vi "simple PID.vi"(4 "lower limit":dbl format="%.2f", 6 "upper limit":dbl format="%.2f", 7 "process variable":dbl format="%.2f", 8 "D":dbl=0.05 format="%.2f", 9 "I":dbl=0.1 format="%.2f", 10 "P":dbl=1.0 format="%.2f", 11 "set point":dbl format="%.2f") -> (3 "output value":dbl format="%.2f")   [LabVIEW 2016]
doc: "This is a simple PID which can be used to control a system. The idea of a PID is to control a system by comparing the set point (the system value you want) to the process variable (the current system value), and adjusting the output value (what you output to the system in an attempt to get the process variable to approach the set point.\n\nThe set point is the value you desire the system to achieve.\n\nThe process variable is the current value of your system, and is usually acquired by an analog input channel of your DAQ device.\n\nP is the Proportional component. This is the amount by which the error gets multiplied. The error is the set point minus the process variable.\n\nI is the Integral component. This is how much the PID output will depend on what has happened in the past.\n\nD is the derivative component. This is how much the PID output will depend on speculation of what will happen in the future.\n\nThe output value is the PID output which is usually generated at an analog output channel of your DAQ device in an attempt to get the process variable equal to the set point.\n\nThe upper limit is the maximum value the PID can output to the system.\n\nThe lower limit is the minimum value the PID can output to the system."
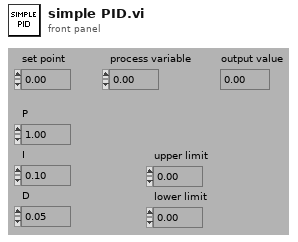
[diagram p1: front panel]
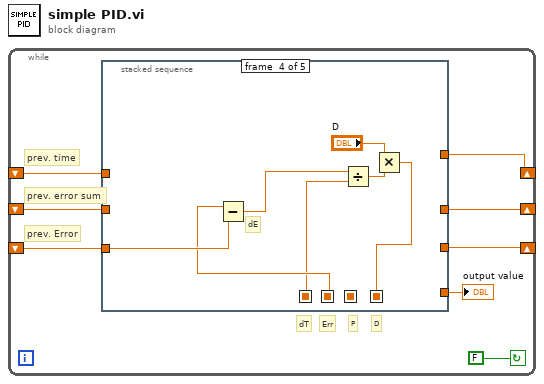
[diagram p0: block diagram]
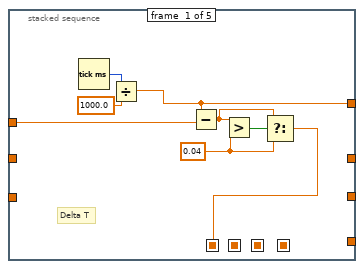
[diagram p2: hidden frame]
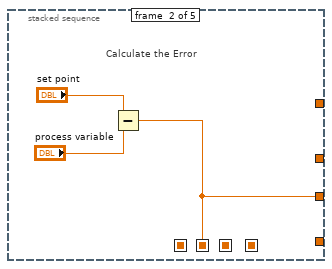
[diagram p3: hidden frame]
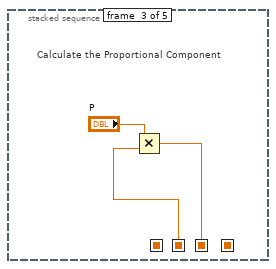
[diagram p4: hidden frame]
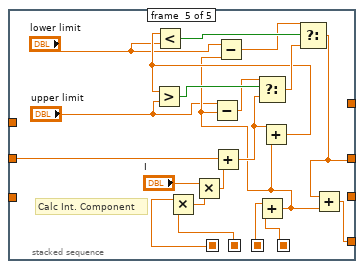
[diagram p5: hidden frame]
diagram:
  n1 = while {
    shift-left: _ -> [w3]
    shift-right: [w4] -> _
    shift-left: _ -> [w6]
    shift-right: [w5] -> _
    shift-left: _ -> [w7]
    shift-right: [w8] -> _
    stop <- FALSE continue-if-true
    # "dT"
    # "Err"
    # "D"
    # "P"
    # "prev. error sum"
    # "prev. time"
    # "prev. Error"
    n2 = stacked-sequence {
      seq-local: [w10 _ _ _ _] -> [_ _ _ w23 w47]
      seq-local: [_ w17 _ _ _] -> [_ _ w21 w28 w48]
      seq-local: [_ _ w20 _ _] -> [_ _ _ _ w43]
      seq-local: [_ _ _ w24 _] -> [_ _ _ _ w42]
      tunnel: [w13 _ _ _ _] -> w8
      tunnel: w7 -> [w16 _ _ _ _]
      tunnel: w6 -> [_ _ _ _ w49]
      tunnel: [_ _ _ _ w36] -> w5
      tunnel: [_ w17 _ _ _] -> w4
      tunnel: w3 -> [_ _ _ w29 _]
      tunnel: [_ _ _ _ w40] -> w2
      frame #0 {
        w9 = 0.04
        # "Delta T"
        n3 = Tick Count (ms)() -> (millisecond timer value=w14:u32)
        n4 = Divide(x=w14, y=1000.0) -> (x/y=w13:dbl)
        n5 = Subtract(x=w13, y=w16) -> (x-y=w11:dbl)
        n6 = Greater?(x=w11, y=w9) -> (0:w12:bool)
        n7 = Select(t=w11, s=w12, f=w9) -> (s? t:f=w10:dbl)
      }
      frame #1 {
        # "Calculate the Error"
        n8 = Subtract(x="set point", y="process variable") -> (x-y=w17:dbl)
      }
      frame #2 {
        # "Calculate the Proportional Component"
        n9 = Multiply(x="P", y=w21) -> (x*y=w20:dbl)
      }
      frame #3 {
        # "dE"
        n10 = Subtract(x=w28, y=w29) -> (x-y=w27:dbl)
        n11 = Divide(x=w27, y=w23) -> (x/y=w26:dbl)
        n12 = Multiply(x="D", y=w26) -> (x*y=w24:dbl)
      }
      frame #4 {
        # "Calc Int. Component"
        n13 = Multiply(x=w47, y=w48) -> (x*y=w46:dbl)
        n14 = Multiply(x="I", y=w46) -> (x*y=w44:dbl)
        n15 = Add(x=w49, y=w44) -> (x+y=w38:dbl)
        n16 = Add(x=w43, y=w42) -> (x+y=w32:dbl)
        n17 = Subtract(x="upper limit", y=w32) -> (x-y=w34:dbl)
        n18 = Subtract(x="lower limit", y=w32) -> (x-y=w33:dbl)
        n19 = Add(x=w38, y=w32) -> (x+y=w35:dbl)
        n20 = Greater?(x=w35, y="upper limit") -> (0:w41:bool)
        n21 = Less?(x=w35, y="lower limit") -> (x < y?=w39:bool)
        n22 = Select(t=w34, s=w41, f=w38) -> (s? t:f=w37:dbl)
        n23 = Select(t=w33, s=w39, f=w37) -> (s? t:f=w36:dbl)
        n24 = Add(x=w36, y=w32) -> (x+y=w40:dbl)
      }
    }
    "output value" <- w2
  }
